vi "PID是否输出判断-子.vi"(1 "数值":dbl) -> (0 "摆角在（-10,10）范围内，开始对电压进行精确的调整":bool)   [LabVIEW 2015]
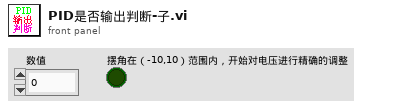
[diagram p1: front panel]
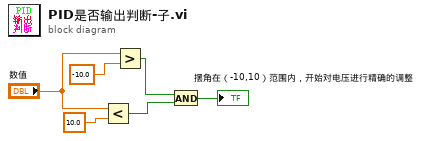
[diagram p0: block diagram]
diagram:
  n1 = Less?(x="数值", y=10.0) -> (x < y?=w4:bool)
  n2 = Greater?(x="数值", y=-10.0) -> (0:w3:bool)
  n3 = And(x=w3, y=w4) -> (x .and. y?=→"摆角在（-10,10）范围内，开始对电压进行精确的调整":bool)
